vi "Router - PXImc Read.vi"(8 "error in (no error)":errorcluster, 9 "Node Properties":T1, 10 "PXImc Cards Properties":T3, 11 "Master Table Ref":refnum<data-value>) -> (0 "error out":errorcluster)   [LabVIEW 2016, in "PXImc Router.lvlib"]
uses:
  PXImc Router.lvlib
  Controls/Router/Router - PXImc Card Properties.ctl
  Controls/Router/Node Block R-W Properties.ctl
  Controls/Router/Block Properties.ctl
  <vilib>/pximc/Acquire Read Region (U8).vi
  <resource>/objmgr/pximc.rc
  <vilib>/pximc/nipximc.lvlib
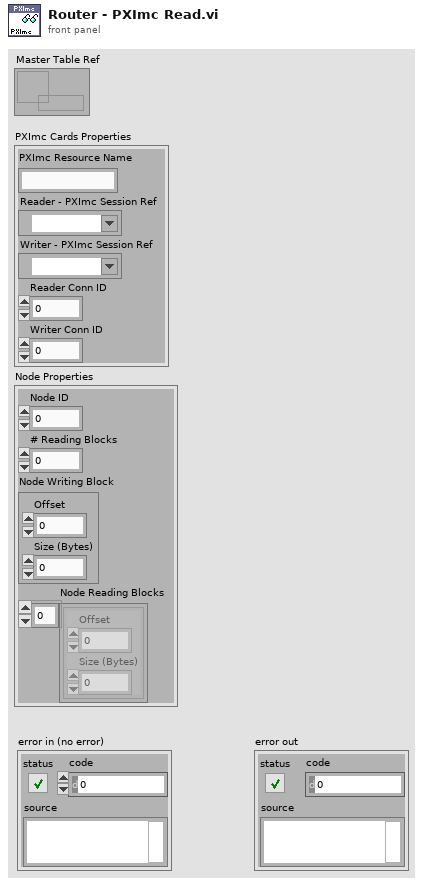
[diagram p1: front panel]
types:
  T1 = typedef "PXImc Router.lvlib/Node Block R-W Properties.ctl" = cluster{"Node ID":u32, "# Reading Blocks":u32, "Node Writing Block":T2, "Node Reading Blocks":T2[]}
  T2 = typedef "PXImc Router.lvlib/Block Properties.ctl" = cluster{"Offset":u32, "Size (Bytes)":u32}
  T3 = typedef "PXImc Router.lvlib/Router - PXImc Card Properties.ctl" = cluster{"PXImc Resource Name":string, "Reader - PXImc Session Ref":refnum<k21>, "Writer - PXImc Session Ref":refnum<k21>, "Reader Conn ID":u16, "Writer Conn ID":u16}
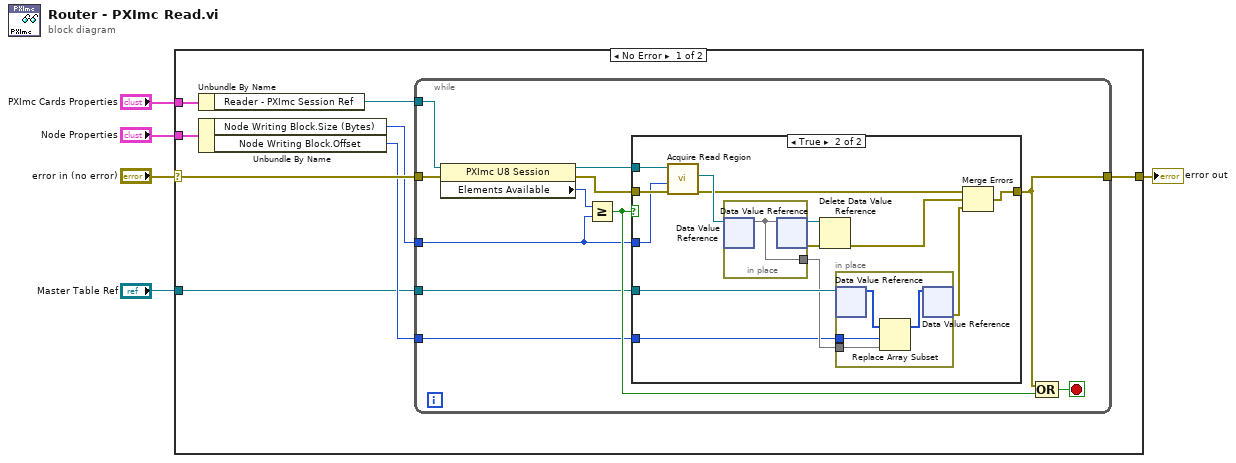
[diagram p0: block diagram]
diagram:
  n1 = case shown="No Error" "error in (no error)" {
    selector: "error in (no error)" -> [w13 w44]
    tunnel: [w12 w44] -> w4
    tunnel: "PXImc Cards Properties" -> [w8 _]
    tunnel: "Node Properties" -> [w7 _]
    tunnel: "Master Table Ref" -> [w6 _]
    frame No Error {
      n2 = Unbundle By Name(w8) -> ("Reader - PXImc Session Ref"=w10:refnum<k21>)
      n3 = Unbundle By Name(w7) -> ("Node Writing Block.Size (Bytes)"=w11:u32, "Node Writing Block.Offset"=w9:u32)
      n4 = while {
        tunnel: w13 -> [w22]
        tunnel: [w18] -> w12
        tunnel: w11 -> [w16]
        tunnel: w10 -> [w17]
        tunnel: w6 -> [w15]
        tunnel: w9 -> [w14]
        stop <- w19 stop-if-true
        n5 = property class="PXImc U8 Session"(reference=w17, error in=w22) -> (reference out=w23:refnum<k21>, error out=w21:errorcluster, "Elements Available"=w24:u64)
        n6 = Greater Or Equal?(x=w24, y=w16) -> (x >= y?=w20:bool)
        n7 = case shown="True" w20 {
          tunnel: w21 -> [w25 w37]
          tunnel: [w25 w31] -> w18
          tunnel: w23 -> [_ w36]
          tunnel: w16 -> [_ w30]
          tunnel: w15 -> [_ w29]
          tunnel: w14 -> [_ w27]
          frame False {
          }
          frame True {
            n8 = call-poly <vilib>:"Acquire Read Region.vi"("error in (no error)"=w37, "number of elements"=w30, "session in"=w36) -> ("error out"=w32:errorcluster, "read region reference"=w38:refnum<data-value>)  [unwired: 5 in, 2 out]
            n9 = in-place {
              in-place-border: [w43] -> w28
              n10 = in-place-dvr #1(w38) -> (w43:u8[])  [unwired: 1 out]
              n11 = in-place-dvr #1(w43) -> (w35:refnum<data-value>, w34:errorcluster)
            }
            n12 = Delete Data Value Reference(data value reference=w35, error in=w34) -> (error out=w33:errorcluster)  [unwired: 1 out]
            n13 = in-place {
              in-place-border: w27 -> [w42]
              in-place-border: w28 -> [w39]
              n14 = in-place-dvr #2(w29) -> (w41:u8[])  [unwired: 1 out]
              n15 = Replace Array Subset(array=w41, new element=w39, index=w42) -> (w40:u8[])
              n16 = in-place-dvr #2(w40) -> (w26:errorcluster)  [unwired: 1 out]
            }
            n17 = Merge Errors(w32, w33, w26) -> (w31:errorcluster)
          }
        }
        n18 = Compound Arithmetic op=OR(w18, w20) -> (w19:bool)
      }
    }
    frame Error {
    }
  }
  "error out" <- w4
